vi "Peer To Peer Reader - 12.8GB (FPGA).vi"() -> ()   [LabVIEW 2023]
uses:
  <vilib>/Platform/TimedLoop/XDataNode/timing_clust.ctl
  <vilib>/Platform/TimedLoop/XDataNode/nitl_modes.ctl
  <vilib>/Platform/TimedLoop/XDataNode/wakeup.ctl
  <vilib>/rvi/Emulation/niFpgaSctlEmulationGetInTimedLoop.vi
  <vilib>/rvi/Emulation/niFpgaEmulationReportErrorSimple.vi
  <vilib>/rvi/Emulation/niFpgaGetClockAttributes.vi
  <vilib>/rvi/Emulation/niFpgaCriticalErrorInLSC.vi
  <vilib>/Platform/TimedLoop/XDataNode/XDataNode.xnode
  <vilib>/rvi/DataTransferAndStorage/Container/XNode/niFpgaContainer.xnode
  <vilib>/Platform/TimedLoop/XDataNode/XDNodeRunTimeDep.lvlib
  <vilib>/rvi/FIFO/Fifo_Resource/nirvififoEmulationP2P.vi
panel:
  out "Data":T1
  out "Data Valid?":bool
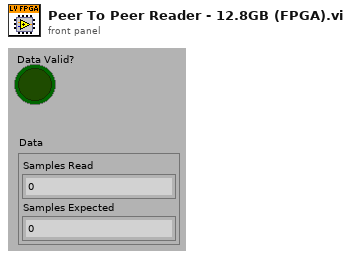
[diagram p1: front panel]
types:
  T1 = cluster{"Samples Read":u64, "Samples Expected":u64}
  T2 = typedef "XDNodeRunTimeDep.lvlib/timing_clust.ctl" = cluster{"Expected End [f-1]":u64, "Actual End [f-1]":u64, "Finished Late? [f-1]":bool, "Expected End [i-1]":u64, "Actual End [i-1]":u64, "Finished Late? [i-1]":bool, "Expected Start [i]":u64, "Actual Start [i]":u64, "Expected Start [f]":u64, "Actual Start [f]":u64, "Source Name":string, "Structure Name":string, "Period":i64, "Deadline":i64, "Offset":i64, "Start":i64, "Priority":i32, "Timeout":i32, "Mode":T3, "Wakeup Reason":T4, "Error":errorcluster, "Source Type":string, "Secondary Source Type":string, "Global End Time":u64, "Global Start Time":u64, "Frame Duration":u64, "Iteration Duration":u64, "Assigned CPU":i32, "I/O Scan Engine Mode":u32}
  T3 = typedef "XDNodeRunTimeDep.lvlib/nitl_modes.ctl" = enum32{"No Change", "Process missed periods, maintain original phase", "Discard missed periods, maintain original phase", "Process missed periods, ignore original phase", "Discard missed periods, ignore original phase"}
  T4 = typedef "XDNodeRunTimeDep.lvlib/wakeup.ctl" = enum32{"Normal", "Aborted", "Asynchronous wakeup", "Timing source error", "Timed loop error", "Timeout"}
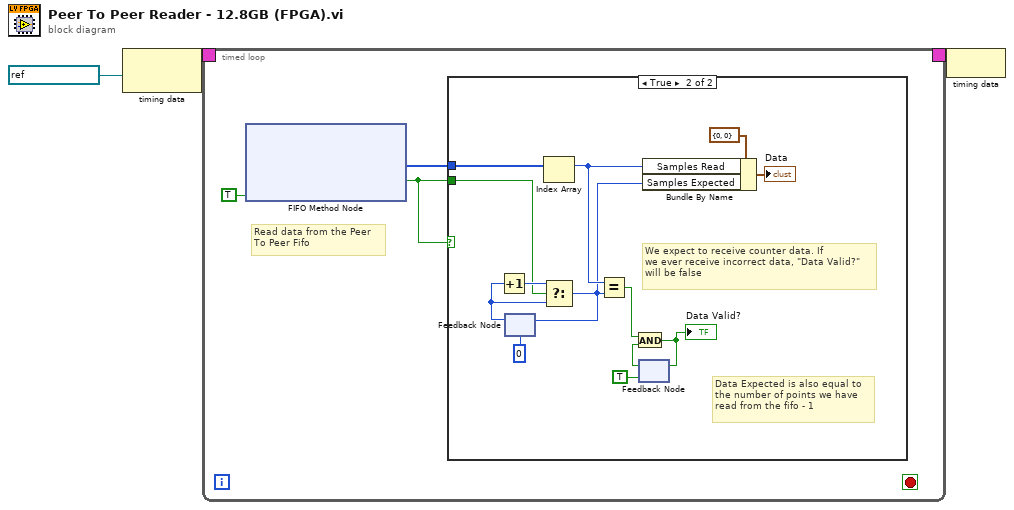
[diagram p0: block diagram]
diagram:
  n1 = node-c288(refnum<k21> "PXIe_Clk100" ("Source Name")) -> (w3:T2)
  n2 = timed-loop {
    timing: w3 -> [_]
    timing-out: [_] -> w2
    stop <- _ stop-if-true
    # "Read data from the Peer \nTo Peer Fifo"
    n3 = xnode ("FIFO Method Node")("Ready for Output"=TRUE) -> ("Element"=w6:u64[], "Output Valid"=w4:bool)  [unwired: 1 in, 1 out]
    n4 = case shown="True" w4 {
      tunnel: w6 -> [_ w17]
      tunnel: w4 -> [_ w11]
      frame False {
      }
      frame True {
        # "We expect to receive counter data. If \nwe ever receive incorrect data, \"Data Valid?\"\nwill be false"
        # "Data Expected is also equal to\nthe number of points we have\nread from the fifo - 1"
        n5 = feedback #1(u64 0 ("Element")) -> (w12:u64)
        n6 = Increment(x=w12) -> (x+1=w13:u64)
        n7 = Index Array(array=w17) -> (element=w8:u64)  [unwired: 1 in]
        n8 = Select(t=w13, s=w11, f=w12) -> (s? t:f=w7:u64)
        n9 = feedback-in #1(w7) -> ()
        n10 = Equal?(x=w8, y=w7) -> (x = y?=w16:bool)
        n11 = feedback #2(TRUE) -> (w15:bool)
        n12 = And(x=w16, y=w15) -> (x .and. y?=w18:bool)
        "Data Valid?" <- w18
        n13 = feedback-in #2(w18) -> ()
        n14 = Bundle By Name(cluster=T1 {"Samples Read"=0, "Samples Expected"=0} ("Data"), "Samples Read"=w8, "Samples Expected"=w7) -> (→"Data":T1)
      }
    }
  }
  n15 = node-c288(w2) -> ()
